vi "Lift.vi"(0 "LiftInput":dbl, 1 "LiftSet":dbl, 2 "LiftSweet":bool) -> ()   [LabVIEW 2017]
uses:
  Phoenix-LabVIEW/Motor Controller/Controls/CTRE_Phoenix_MotorControl_ControlMode.ctl
  Robot Global Data.vi
  <vilib>/addons/control/pid/pid.llb/PID (DBL).vi
  <vilib>/addons/control/pid/NI_PID_pid.lvlib
panel:
  in  "G":dbl=-0.2
  in  "Lift PID":T1={"proportional gain (Kc)"=-3.3, "integral time (Ti, min)"=0.0, "derivative time (Td, min)"=0.0} {"derivative time (Td, min)" format="%.3f"; "integral time (Ti, min)" format="%.3f"; "proportional gain (Kc)" format="%.3f"}
  out "LiftPosActual":dbl format="%#_13g"
  in  "LiftMax":dbl=0.95
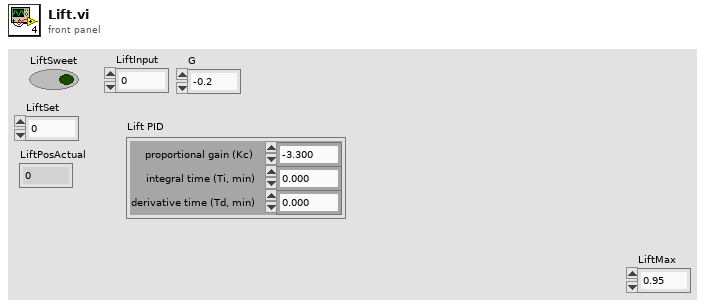
[diagram p1: front panel]
types:
  T1 = cluster{"proportional gain (Kc)":dbl, "integral time (Ti, min)":dbl, "derivative time (Td, min)":dbl}
  T2 = typedef "CTRE_Phoenix_MotorControl_ControlMode.ctl" = u16
  T3 = typedef "WPI_MotorControlDeviceRef.ctl" = cluster{"DeviceStatus":errorcluster, "Type":T4, "PWM":cluster{"PWM Channel":T5, "DeadBand":T6}, "CAN":cluster{"Device Number":u8, "SetOutput VI Ref":variant, "GetOutput VI Ref":variant, "Enable VI Ref":variant, "Disable VI Ref":variant, "Data":variant}, "Invert":bool, "DIO PWM":cluster{"PWM \"Enable\" Channel":T5, "DIOChannel":T7, "PWM Rate":dbl}}
  T4 = typedef "WPI_MotorControlType.ctl" = enum16{"PWM", "CAN", "DIO PWM"}
  T5 = typedef "FPGA_DIOPWMChannel.ctl" = enum8{"PWM 0", "PWM 1", "PWM 2", "PWM 3", "PWM 4", "PWM 5", "PWM 6", "PWM 7", "PWM 8", "PWM 9", "PWM MXP 0", "PWM MXP 1", "PWM MXP 2", "PWM MXP 3", "PWM MXP 4", "PWM MXP 5", "PWM MXP 6", "PWM MXP 7", "PWM MXP 8", "PWM MXP 9", "Invalid"}
  T6 = typedef "WPI_PWMDeadband.ctl" = cluster{"Name":string, "maxPositivePwm":i32, "minPositivePwm":i32, "centerPwm":i32, "maxNegativePwm":i32, "minNegativePwm":i32, "angularRange":u16}
  T7 = typedef "FPGA_DIOChannel.ctl" = enum8{"DIO 0", "DIO 1", "DIO 2", "DIO 3", "DIO 4", "DIO 5", "DIO 6", "DIO 7", "DIO 8", "DIO 9", "DIO MXP 0", "DIO MXP 1", "DIO MXP 2", "DIO MXP 3", "DIO MXP 4", "DIO MXP 5", "DIO MXP 6", "DIO MXP 7", "DIO MXP 8", "DIO MXP 9", "DIO MXP 10", "DIO MXP 11", "DIO MXP 12", "DIO MXP 13", "DIO MXP 14", "DIO MXP 15", "SPI Port CS1", "SPI Port CS2", "SPI Port CS3", "SPI Port MISO", "SPI Port MOSI", "Invalid"}
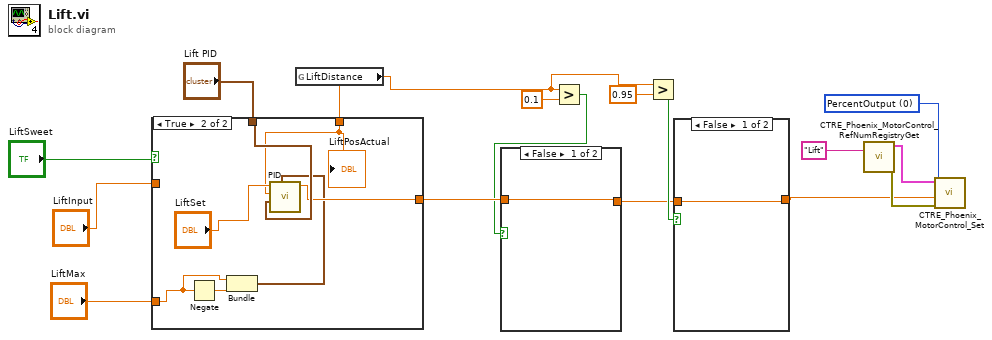
[diagram p0: block diagram]
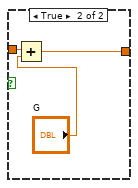
[diagram p2: hidden frame]
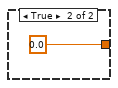
[diagram p3: hidden frame]
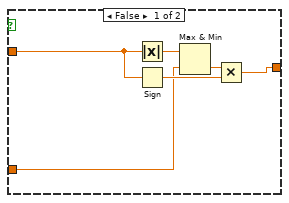
[diagram p4: hidden frame]
diagram:
  w14 = T2 0 items=["PercentOutput"=0, "Position"=1, "Velocity"=2, "Current"=3, "Follower"=5, "MotionProfile"=6, "MotionMagic"=7, "MotionMagicArc"=8, "MotionProfileArc"=10, "Disabled"=15] ("Control Mode")
  n1 = global read "Robot Global Data.vi" "LiftDistance"() -> (w6:dbl)
  n2 = case shown="True" "LiftSweet" {
    tunnel: [w19 w28] -> w7
    tunnel: "Lift PID" -> [_ w29]
    tunnel: "LiftInput" -> [w18 _]
    tunnel: "LiftMax" -> [w17 w26]
    tunnel: w6 -> [_ w23]
    frame False {
      n3 = Absolute Value(x=w18) -> (abs(x)=w20:dbl)
      n4 = Sign(1:w18) -> (0:w21:dbl)
      n5 = Max & Min(x=w20, y=w17) -> (min(x,y)=w22:dbl)  [unwired: 1 out]
      n6 = Multiply(x=w22, y=w21) -> (x*y=w19:dbl)
    }
    frame True {
      n7 = Negate(x=w26) -> (-x=w27:dbl)
      n8 = Bundle("LiftMax"=w26, w27) -> (w25:cluster{"LiftMax":dbl, dbl})  [unwired: 1 in]
      n9 = call-poly <vilib>:"PID.vi"("output range"=w25, "PID gains"=w29, "process variable"=w23, "setpoint"="LiftSet") -> ("output"=w28:dbl)  [unwired: 6 in, 1 out]
      "LiftPosActual" <- w23
    }
  }
  n10 = Greater?(x=w6, y=0.1) -> (0:w1:bool)
  n11 = case shown="False" w1 {
    tunnel: w7 -> [w30 w33]
    tunnel: [w30 w31] -> w2
    frame False {
    }
    frame True {
      n12 = Add(x=w33, y="G") -> (x+y=w31:dbl)
    }
  }
  n13 = Greater?(x=w6, y=0.95) -> (0:w4:bool)
  n14 = case shown="False" w4 {
    tunnel: [w34 0.0] -> w3
    tunnel: w2 -> [w34 _]
    frame False {
    }
    frame True {
    }
  }
  n15 = call "CTRE_Phoenix_MotorControl_RefNumRegistryGet.vi"("refnum name"="Lift") -> ("error out"=w13:errorcluster, "PhoenixMotorControlDevRef"=w15:T3)  [unwired: 9 in]
  n16 = call "CTRE_Phoenix_MotorControl_Set.vi"("error in (no error)"=w13, "Output"=w3, "Control Mode"=w14, "PhoenixMotorControlDevRef"=w15) -> ()  [unwired: 6 in, 2 out]
